vi "IO_MFA_AIN_Read_AnalogueInput1.vi"() -> (3 "ADC":sgl format="%.2f")   [LabVIEW 2018]
panel:
  out "error ADC":errorcluster
  out "AAABuild":i32
  in  "MintController":refnum<k7>(container)
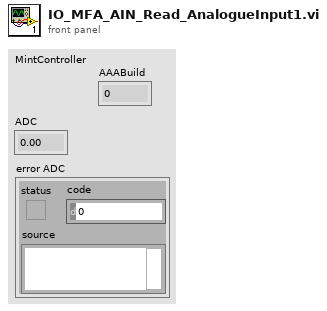
[diagram p1: front panel]
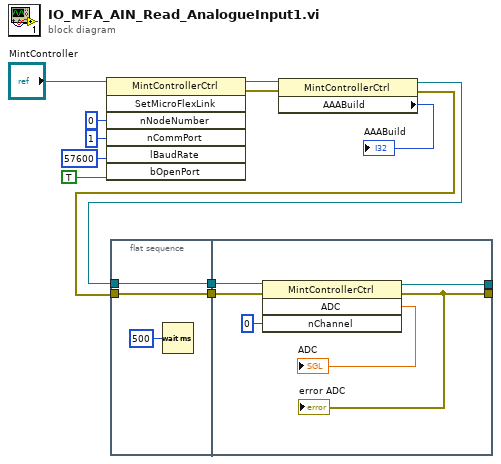
[diagram p0: block diagram]
diagram:
  n1 = invoke class="MintControllerCtrl" method="SetMicroFlexLink"(reference="MintController", "nNodeNumber"=i16 0, "nCommPort"=i16 1, "lBaudRate"=57600, "bOpenPort"=TRUE) -> (reference out=w12:refnum<k7>, error out=w6:errorcluster)  [unwired: 2 in, 5 out]
  n2 = flat-sequence {
    tunnel: [w15] -> w4
    tunnel: [w13] -> w3
    tunnel: w2 -> [w15]
    tunnel: w1 -> [w13]
    tunnel: w4 -> [w21]
    tunnel: w3 -> [w20]
    tunnel: [w18] -> _
    tunnel: [w17] -> _
    frame #0 {
      n3 = Wait (ms)(milliseconds to wait=u32 500) -> ()  [unwired: 1 out]
    }
    frame #1 {
      n4 = invoke class="MintControllerCtrl" method="ADC"(reference=w20, error in=w21, "nChannel"=i16 0) -> (reference out=w17:refnum<k7>, error out=w18:errorcluster, "ADC"=→"ADC":sgl)  [unwired: 1 in, 1 out]
      "error ADC" <- w18
    }
  }
  n5 = property class="MintControllerCtrl"(reference=w12, error in=w6) -> (reference out=w1:refnum<k7>, error out=w2:errorcluster, "AAABuild"=→"AAABuild":i32)
